vi "LINC Get Application Path.vi"(8 "error in (no error)":errorcluster) -> (0 "error out":errorcluster, 3 "application path":path)   [LabVIEW 2018, in "STEPkgDriver_LINC.lvlib"]
uses:
  STEPkgDriver_LINC.lvlib
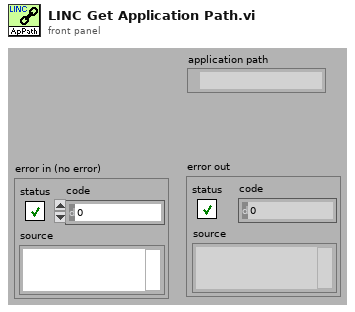
[diagram p1: front panel]
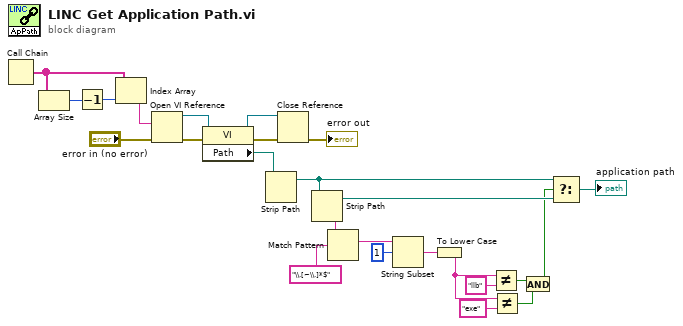
[diagram p0: block diagram]
diagram:
  n1 = Call Chain() -> (call chain=w25:string[])
  n2 = Array Size(array=w25) -> (size(s)=w24:i32)
  n3 = Decrement(x=w24) -> (x-1=w23:i32)
  n4 = Index Array(array=w25, index=w23) -> (element=w22:string)
  n5 = Open VI Reference(vi path=w22, error in (no error)="error in (no error)") -> (vi reference=w21:refnum<vi>, error out=w20:errorcluster)  [unwired: 4 out]
  n6 = property class="VI"(reference=w21, error in=w20) -> (reference out=w18:refnum<vi>, error out=w19:errorcluster, "Path"=w17:path)
  n7 = Strip Path(path=w17) -> (stripped path=w10:path)  [unwired: 1 out]
  n8 = Close Reference(reference=w18, error in (no error)=w19) -> (error out=→"error out":errorcluster)
  n9 = Strip Path(path=w10) -> (stripped path=w9:path, name=w12:string)
  n10 = Match Pattern(string=w12, regular expression="\\.[~\\.]*$") -> (match substring=w13:string)  [unwired: 4 out]
  n11 = String Subset(string=w13, offset (0)=1) -> (substring=w14:string)  [unwired: 1 out]
  n12 = To Lower Case(string=w14) -> (all lower case string=w4:string)
  n13 = Not Equal?(x=w4, y="llb") -> (x != y?=w7:bool)
  n14 = Not Equal?(x=w4, y="exe") -> (x != y?=w6:bool)
  n15 = And(x=w7, y=w6) -> (x .and. y?=w5:bool)
  n16 = Select(t=w10, s=w5, f=w9) -> (s? t:f=→"application path":path)
